vi "Matrix_Ident.vi"(11 "Size":i32) -> (0 "Error":bool, 3 "output matrix":T1)   [LabVIEW 2019, in "Trajectory_Library.lvlib"]
doc: "Creates the identity matrix of the given dimension.\n \nInputs:\n - size -- The dimension of the desired matrix.\n\nOutputs:\n - output matrix -- The DxD identity matrix.\n - error -- If TRUE, an error occured."
uses:
  Trajectory_Library.lvlib
  <vilib>/Analysis/Matrix/Datatypes/RealMatrix.ctl
  <vilib>/Analysis/7linalg.llb/Create Special Real Matrix.vi
  <vilib>/Analysis/NI_AALPro.lvlib
  <vilib>/Analysis/Matrix/NI_Matrix.lvlib
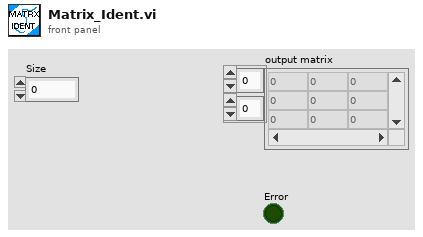
[diagram p1: front panel]
types:
  T1 = typedef "NI_Matrix.lvlib/RealMatrix.ctl" = dbl[][]
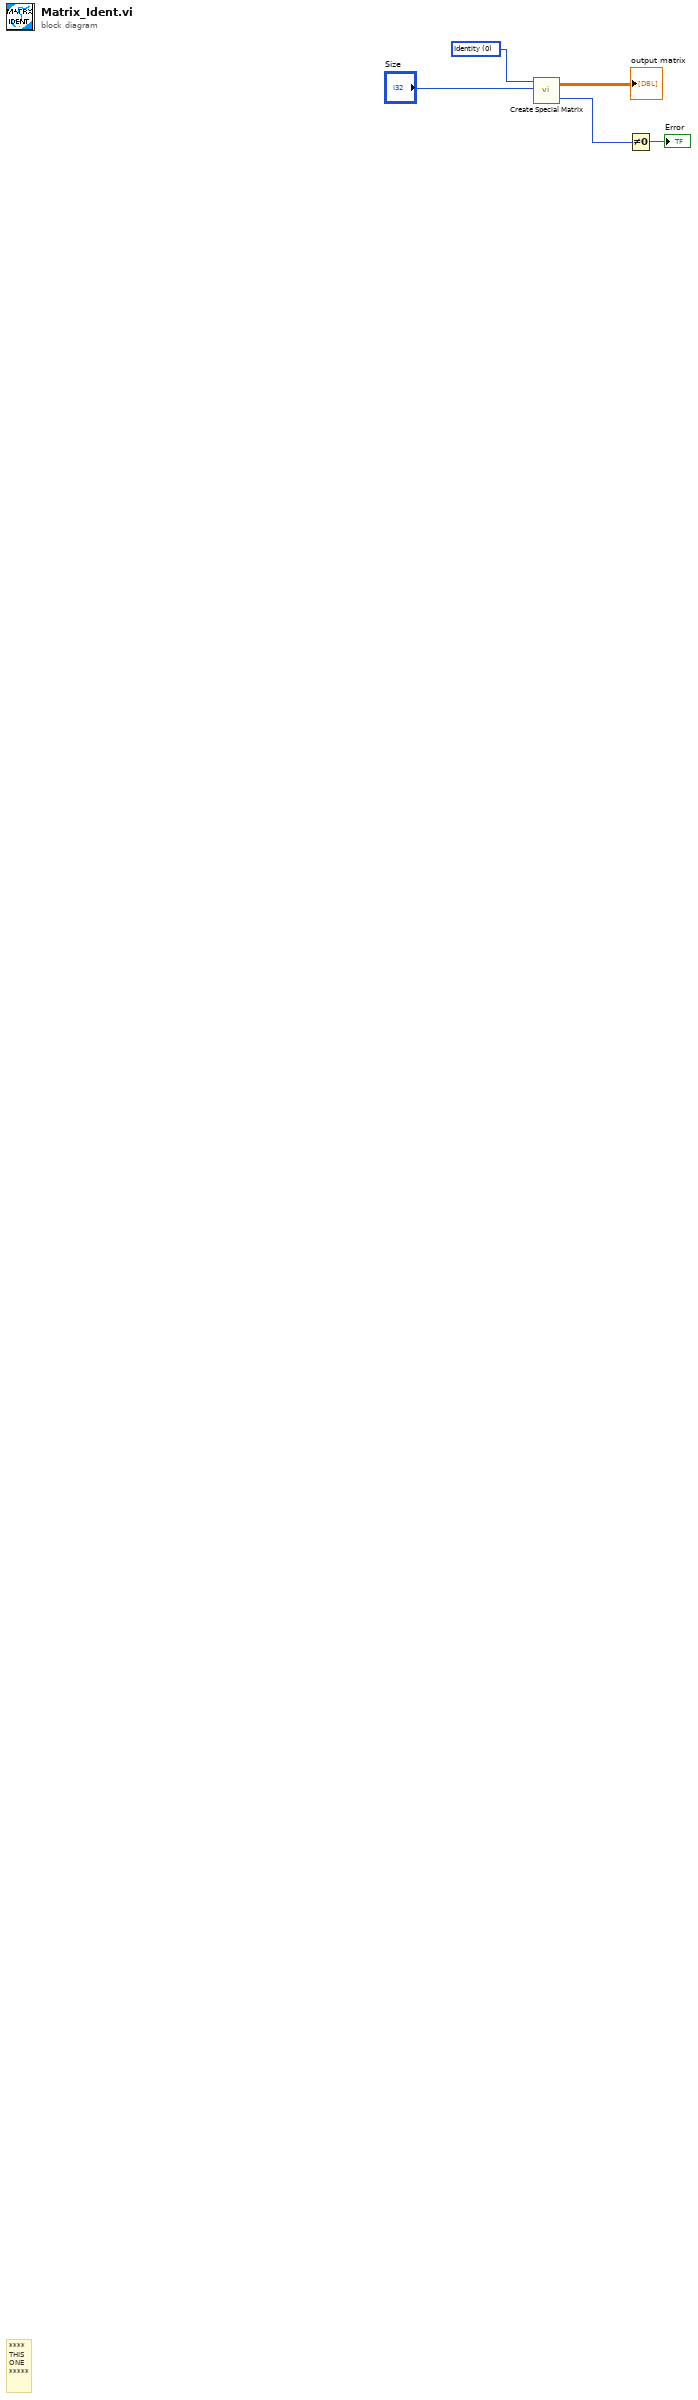
[diagram p0: block diagram]
diagram:
  w5 = 0 items=["Identity", "Diagonal", "Toeplitz", "Vandermonde", "Companion", "Hankel", "Hadamard", "Wilkinson", "Hilbert", "Inverse Hilbert", "Rosser", "Pascal"] ("matrix type")
  # "****\nTHIS\nONE\n*****"
  n1 = call-poly <vilib>:"Create Special Matrix.vi"("matrix type"=w5, "matrix size"="Size") -> ("Special Matrix"=→"output matrix":T1, "error"=w1:i32)  [unwired: 3 in]
  n2 = Not Equal To 0?(x=w1) -> (x != 0?=→"Error":bool)
